vi "LT.vi"(1 "Ctl Refnum 2":refnum<vi>, 2 "Ctl Refnum":refnum<vi>, 3 "Function (0: Cp-D)":u16(ring) items=["Cp-D", "Cp-Q", "Cp-G", "Cp-Rp", "Cs-D", "Cs-Q", "Cs-Rs", "Lp-D", "Lp-Q", "Lp-G", "Lp-Rp", "Lp-Rdc", "Ls-D", "Ls-Q", "Ls-Rs", "Ls-Rdc", "R-X", "Z-thd", "Z-thr", "G-B", "Y-thd", "Y-thr", "Vdc-Idc"], 8 "error in (no error)":errorcluster caption="错误输入（无错误）", 9 "Cluster 3":T1={"客户仪器地址"="USB0::0x0471::0x2826::QF71600867::INSTR", "低温地址"="COM3"}, 10 "Cluster":T2={"开始温度"=22.54, "变温速率"=3.0, "结束温度"=50.0, "簇"={"测试频率"=100000.0, "测试频率 2"=100000.0, "测试频率 3"=100000.0, "测试频率 4"=100000.0}}, 11 "Cluster 2":cluster{"文本数据路径：":path, "表格数据路径： ":path}={"文本数据路径："=path "C:/Users/shipeng/Desktop/LT Dielectric measurement", "表格数据路径： "=path "C:/Users/shipeng/Desktop/LT Dielectric measurement"}) -> (0 "错误输出":cluster{"状态":bool, "代码":i32, "源":string})   [LabVIEW 2017]
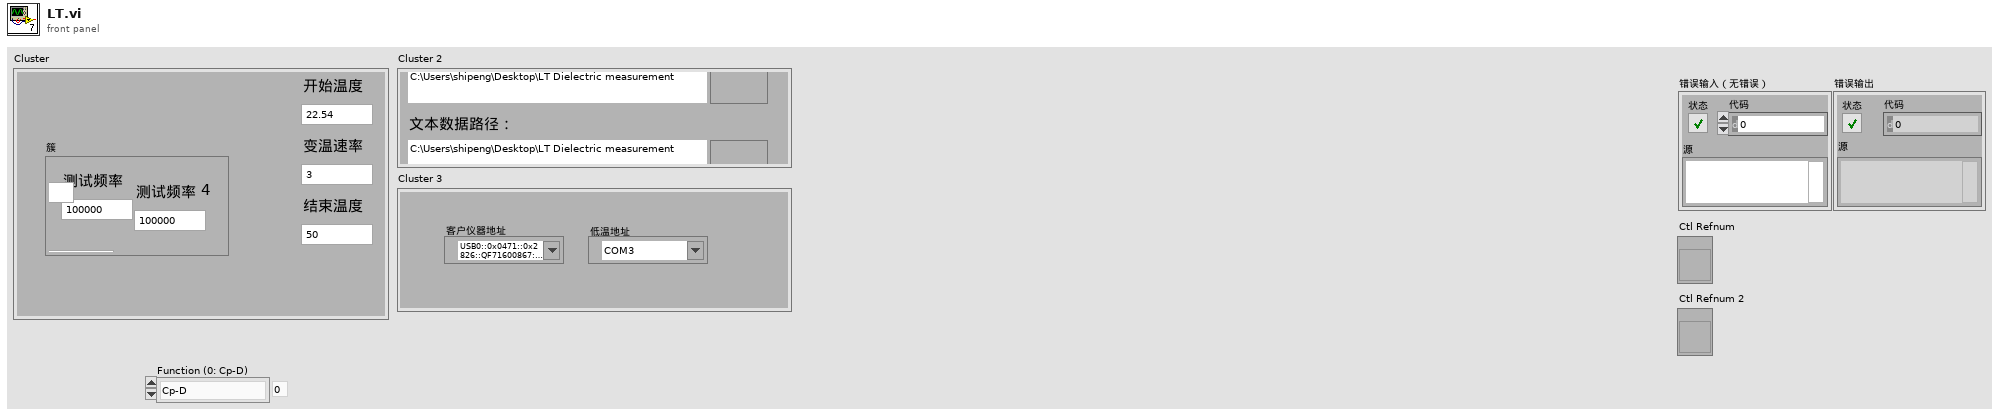
[diagram p1: front panel]
types:
  T1 = cluster{"客户仪器地址":refnum<visa-resource-name>, "低温地址":refnum<visa-resource-name>}
  T2 = cluster{"开始温度":dbl, "变温速率":dbl, "结束温度":dbl, "簇":cluster{"测试频率":dbl, "测试频率 2":dbl, "测试频率 3":dbl, "测试频率 4":dbl}}
  T3 = enum16{"open", "replace", "create", "open or create", "replace or create", "replace or create with confirmation"}
  T4 = cluster{"测试频率":dbl, "测试频率 2":dbl, "测试频率 3":dbl, "测试频率 4":dbl}
  T5 = cluster{"客户仪器地址":refnum<visa-resource-name>, "低温地址":refnum<visa-resource-name>, "refnum out":refnum<file>, "簇":cluster{"测试频率":dbl, "测试频率 2":dbl, "测试频率 3":dbl, "测试频率 4":dbl}, "error out":errorcluster, "结束温度":dbl, "开始温度":dbl}
  T6 = cluster{"Array":string[][], "error out":errorcluster}
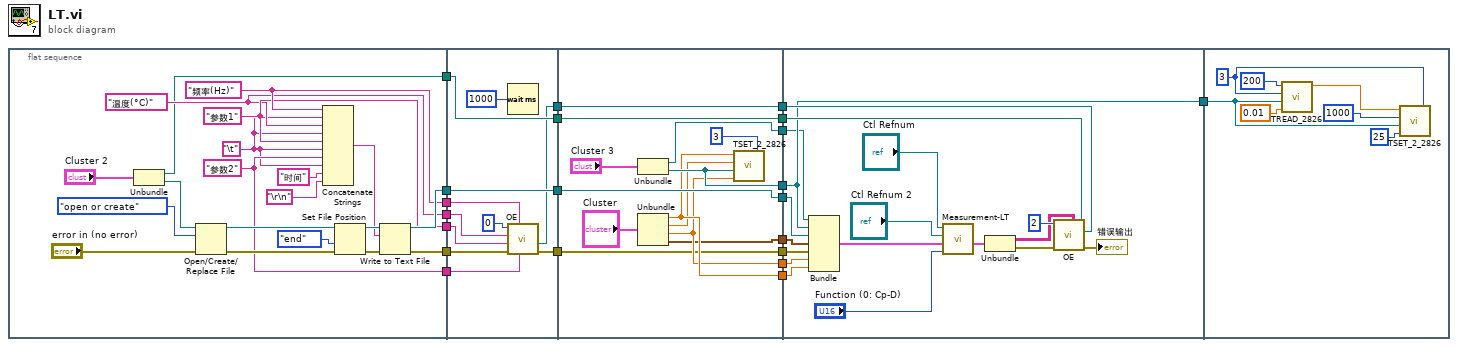
[diagram p0: block diagram]
diagram:
  n1 = flat-sequence {
    tunnel: [w34] -> w21
    tunnel: [w33] -> w20
    tunnel: [w31] -> w17
    tunnel: [w30] -> w16
    tunnel: [w29] -> w15
    tunnel: [w28] -> w14
    tunnel: [w22] -> w10
    tunnel: w21 -> [w51]
    tunnel: [w51] -> w5
    tunnel: w20 -> [w44]
    tunnel: w17 -> [w48]
    tunnel: w16 -> [w45]
    tunnel: w15 -> [w46]
    tunnel: w14 -> [w47]
    tunnel: [w43] -> w4
    tunnel: [w50] -> w3
    tunnel: w10 -> [w50]
    tunnel: [w42] -> w2
    tunnel: w5 -> [w64]
    tunnel: [w64] -> w19
    tunnel: [w54] -> w18
    tunnel: w4 -> [w63]
    tunnel: [w63] -> w13
    tunnel: [w57] -> w12
    tunnel: [w62] -> w11
    tunnel: w3 -> [w62]
    tunnel: [w61] -> w9
    tunnel: [w58] -> w8
    tunnel: [w60] -> w6
    tunnel: w2 -> [w54]
    tunnel: [w53] -> w1
    tunnel: w19 -> [w82]
    tunnel: w18 -> [w83]
    tunnel: w13 -> [w80]
    tunnel: w12 -> [w81]
    tunnel: w11 -> [w79]
    tunnel: w9 -> [w69]
    tunnel: w8 -> [w70]
    tunnel: [w69] -> w7
    tunnel: w6 -> [w68]
    tunnel: w1 -> [w67]
    tunnel: w7 -> [w85]
    frame #0 {
      w30 = "参数2" ("字符串")
      w29 = "参数1" ("字符串")
      w28 = "温度(°C)" ("字符串")
      w27 = "\t"
      w31 = "频率(Hz)" ("字符串")
      n2 = Unbundle("Cluster 2") -> ("文本数据路径："=w22:path, "表格数据路径："=w23:path)
      n3 = Open/Create/Replace File(file path (use dialog)=w23, error in="error in (no error)", operation (0:open)=T3."open or create" ("操作(0:open)")) -> (refnum out=w39:refnum<file>, error out=w36:errorcluster)  [unwired: 4 out]
      n4 = Concatenate Strings(w31, w27, w28, w27, w29, w27, w30, w27, "时间" ("字符串"), "\r\n") -> (w35:string)
      n5 = Set File Position(refnum=w39, from (0:start)=enum16{"start", "end", "current"}."end" ("自（0:起始）"), error in=w36) -> (refnum out=w40:refnum<file>, error out=w41:errorcluster)  [unwired: 1 out]
      n6 = Write to Text File(file (use dialog)=w40, text=w35, error in=w41) -> (refnum out=w34:refnum<file>, error out=w33:errorcluster)  [unwired: 2 out]
    }
    frame #1 {
      n7 = Wait (ms)(milliseconds to wait=u32 1000 ("等待时间（毫秒）")) -> ()  [unwired: 1 out]
      n8 = call "OE.vi"("String 4"=w45, "String"=w48, "error in (no error)"=w44, "String 3"=w46, "String 2"=w47, "Numeric"=0) -> ("error out"=w42:errorcluster, "report out"=w43:refnum<class "NI_report.lvclass">)  [unwired: 3 in, 1 out]
    }
    frame #2 {
      n9 = Unbundle("Cluster 3") -> ("客户仪器地址"=w53:refnum<visa-resource-name>, "低温地址"=w61:refnum<visa-resource-name>)
      n10 = Unbundle("Cluster") -> ("开始温度"=w60:dbl, "变温速率"=w59:dbl, "结束温度"=w58:dbl, "簇"=w57:T4)
      n11 = call "TSET_2_2826.vi"("Address No."=i8 3, "T-Ending, C"=w58, "VISA resource name"=w61, "cooling/heating rate, C/min"=w59, "T-Starting, C"=w60) -> ()
    }
    frame #3 {
      n12 = Bundle("客户仪器地址"=w67, "低温地址"=w69, "refnum out"=w82, "簇"=w81, "error out"=w83, "结束温度"=w70, "开始温度"=w68) -> (w76:T5)  [unwired: 1 in]
      n13 = call "Measurement-LT.vi"("Function (0: Cp-D)"="Function (0: Cp-D)", "Cluster 2"=w76, "Ctl Refnum 2"="Ctl Refnum 2", "Ctl Refnum"="Ctl Refnum") -> ("Cluster"=w75:T6)  [unwired: 7 in]
      n14 = Unbundle(w75) -> ("Array"=w73:string[][], "error out"=w74:errorcluster)
      n15 = call "OE.vi"("report in"=w80, "表格数据路径："=w79, "Array"=w73, "error in (no error)"=w74, "Numeric"=2) -> ("error out"=→"错误输出":errorcluster)  [unwired: 4 in, 2 out]
    }
    frame #4 {
      w87 = i8 3 ("Address No.")
      n16 = call "TREAD_2826.vi"("Unknown Param 2"=0.01, "VISA resource name"=w85, "Address No."=w87, "Unknown Param"=200) -> ("PV"=w84:dbl)  [unwired: 3 out]
      n17 = call "TSET_2_2826.vi"("Address No."=w87, "T-Ending, C"=25, "VISA resource name"=w85, "cooling/heating rate, C/min"=1000, "T-Starting, C"=w84) -> ()
    }
  }
